vi "Set DS Alert Active Status.vi"(8 "error in (no error)":errorcluster, 11 "handle":i64) -> (0 "error out":errorcluster)   [LabVIEW 2026, in "MrcLib.lvlib"]
doc: "Make the referenced Alert active or inactive."
uses:
  MrcLib.lvlib
panel:
  in  "active":bool
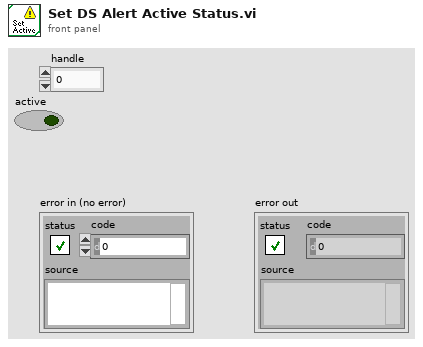
[diagram p1: front panel]
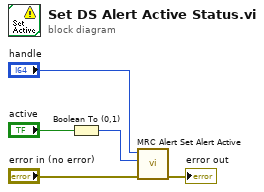
[diagram p0: block diagram]
diagram:
  n1 = Boolean To (0,1)(Boolean="active") -> (0, 1=w1:i16)
  n2 = call "MRC Alert Set Alert Active.vi"("error in (no error)"="error in (no error)", "active"=w1, "handle"="handle") -> ("error out"=→"error out":errorcluster)  [unwired: 8 in]
